vi "Read to Char.vi"(6 "Char":string, 8 "error in (no error)":errorcluster, 11 "VISA resource name in":refnum<visa-resource-name>) -> (0 "error out":errorcluster, 2 "Response":string, 3 "VISA resource name":refnum<visa-resource-name>)   [LabVIEW 2024, in "CTIPicoVISA.lvlib"]
uses:
  CTIPicoVISA.lvlib
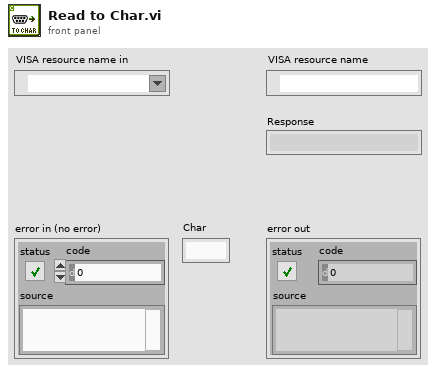
[diagram p1: front panel]
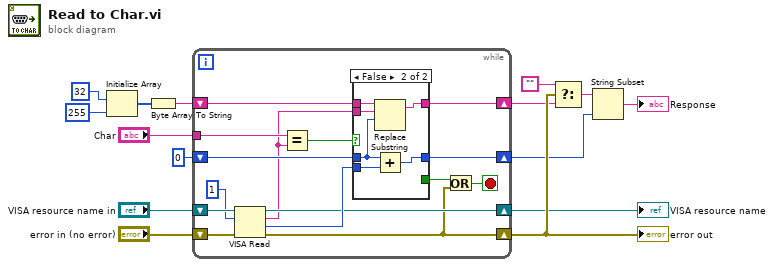
[diagram p0: block diagram]
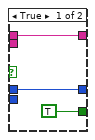
[diagram p2: hidden frame]
diagram:
  n1 = Initialize Array(u8 32 ("element"), 255 ("dimension size")) -> (w12:u8[])
  n2 = Byte Array To String(unsigned byte array=w12) -> (string=w11:string)
  n3 = while {
    shift-right: [w20] -> w15
    shift-left: "error in (no error)" -> [w29]
    shift-right: [w21] -> w1
    shift-left: "VISA resource name in" -> [w30]
    shift-right: [w24] -> w10
    shift-left: w11 -> [w27]
    shift-right: [w25] -> w7
    shift-left: u32 0 -> [w26]
    tunnel: "Char" -> [w18]
    stop <- w22 stop-if-true
    n4 = VISA Read(VISA resource name=w30, byte count=u32 1, error in (no error)=w29) -> (VISA resource name out=w21:refnum<visa-resource-name>, read buffer=w16:string, return count=w23:u32, error out=w20:errorcluster)
    n5 = Equal?(x=w18, y=w16) -> (x = y?=w17:bool)
    n6 = case shown="False" w17 {
      tunnel: w27 -> [w33 w39]
      tunnel: w26 -> [w32 w38]
      tunnel: [w32 w37] -> w25
      tunnel: [w33 w36] -> w24
      tunnel: w23 -> [_ w35]
      tunnel: [TRUE _] -> w19
      tunnel: w16 -> [_ w34]
      frame True {
      }
      frame False {
        n7 = Replace Substring(3:w38, 4:w34, 5:w39) -> (1:w36:string)  [unwired: 1 in, 1 out]
        n8 = Add(x=w38, y=w35) -> (x+y=w37:u32)
      }
    }
    n9 = Or(x=w19, y=w20) -> (x .or. y?=w22:bool)
  }
  "VISA resource name" <- w1
  "error out" <- w15
  n10 = Select(t="", s=w15, f=w10) -> (s? t:f=w8:string)
  n11 = String Subset(string=w8, length (rest)=w7) -> (substring=→"Response":string)  [unwired: 1 in]
